vi "1_1.vi"() -> ()   [LabVIEW 2010]
panel:
  out "sin1(x)=":dbl
  out "ms 2":u32
  out "s 2":dbl
  out "s 1":dbl
  out "ms 1":u32
  out "sin2(x)=":dbl
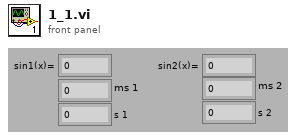
[diagram p1: front panel]
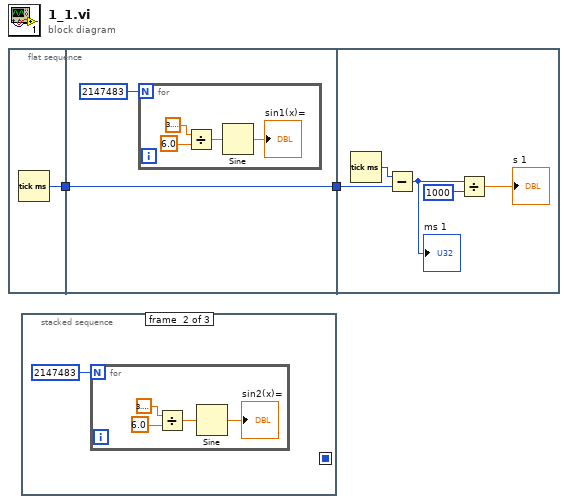
[diagram p0: block diagram]
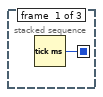
[diagram p2: hidden frame]
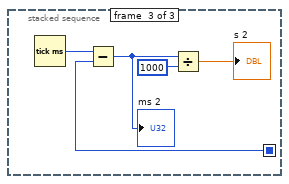
[diagram p3: hidden frame]
diagram:
  n1 = flat-sequence {
    tunnel: [w3] -> w2
    tunnel: w2 -> [w5]
    tunnel: [w5] -> w1
    tunnel: w1 -> [w13]
    frame #0 {
      n2 = Tick Count (ms)() -> (millisecond timer value=w3:u32)
    }
    frame #1 {
      n3 = for {
        N: 2147483 -> [_]
        n4 = Divide(x=3.141592653589793, y=6.0) -> (x/y=w7:dbl)
        n5 = Sine(x=w7) -> (sin(x)=→"sin1(x)=":dbl)
      }
    }
    frame #2 {
      n6 = Tick Count (ms)() -> (millisecond timer value=w14:u32)
      n7 = Subtract(x=w14, y=w13) -> (x-y=w12:u32)
      "ms 1" <- w12
      n8 = Divide(x=w12, y=u32 1000) -> (x/y=→"s 1":dbl)
    }
  }
  n9 = stacked-sequence {
    seq-local: [w15 _ _] -> [_ _ w21]
    frame #0 {
      n10 = Tick Count (ms)() -> (millisecond timer value=w15:u32)
    }
    frame #1 {
      n11 = for {
        N: 2147483 -> [_]
        n12 = Divide(x=3.141592653589793, y=6.0) -> (x/y=w18:dbl)
        n13 = Sine(x=w18) -> (sin(x)=→"sin2(x)=":dbl)
      }
    }
    frame #2 {
      n14 = Tick Count (ms)() -> (millisecond timer value=w25:u32)
      n15 = Subtract(x=w25, y=w21) -> (x-y=w24:u32)
      "ms 2" <- w24
      n16 = Divide(x=w24, y=u32 1000) -> (x/y=→"s 2":dbl)
    }
  }
